vi "calcReturnTime.vi"(3 "Galvo obj array":refnum<class "Galvonometer.lvclass">[](array[class])=[refnum, refnum], 4 "Scan in":refnum<class "Scan.lvclass">, 5 "Camera in":refnum<class "Camera.lvclass">) -> (1 "Delay A":dbl, 2 "Inactive A":dbl)   [LabVIEW 2017]
uses:
  classes/Scans/Scan.lvclass
  classes/HardwareObjects/Camera/Camera.lvclass
  classes/HardwareObjects/Galvonometer/Galvonometer.lvclass
  classes/Scans/Scan.lvclass/Scan.ctl
  classes/HardwareObjects/Camera/Camera.lvclass/Camera.ctl
  classes/HardwareObjects/Galvonometer/Galvonometer.lvclass/Galvonometer.ctl
  classes/HardwareObjects/Galvonometer/Read Output Scale Factor (V_degrees).vi
  classes/HardwareObjects/Galvonometer/Read Max Scan Angle (degrees).vi
  classes/HardwareObjects/Camera/Read Max Frequency (kHz).vi
  classes/Scans/Read Scan Angle (degrees).vi
  classes/Scans/Read X FOV (degrees).vi
  classes/Scans/Read Y FOV (degrees).vi
  classes/Scans/Read Bidirectional.vi
panel:
  out "Return distance (°)":dbl=5.830951894845301
  out "Return time (s)":dbl
  out "Max angular velocity (°/s)":i32=8750
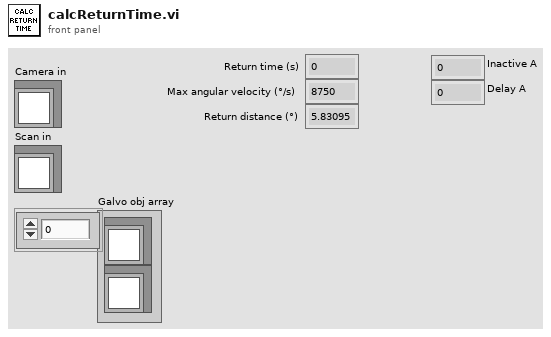
[diagram p1: front panel]
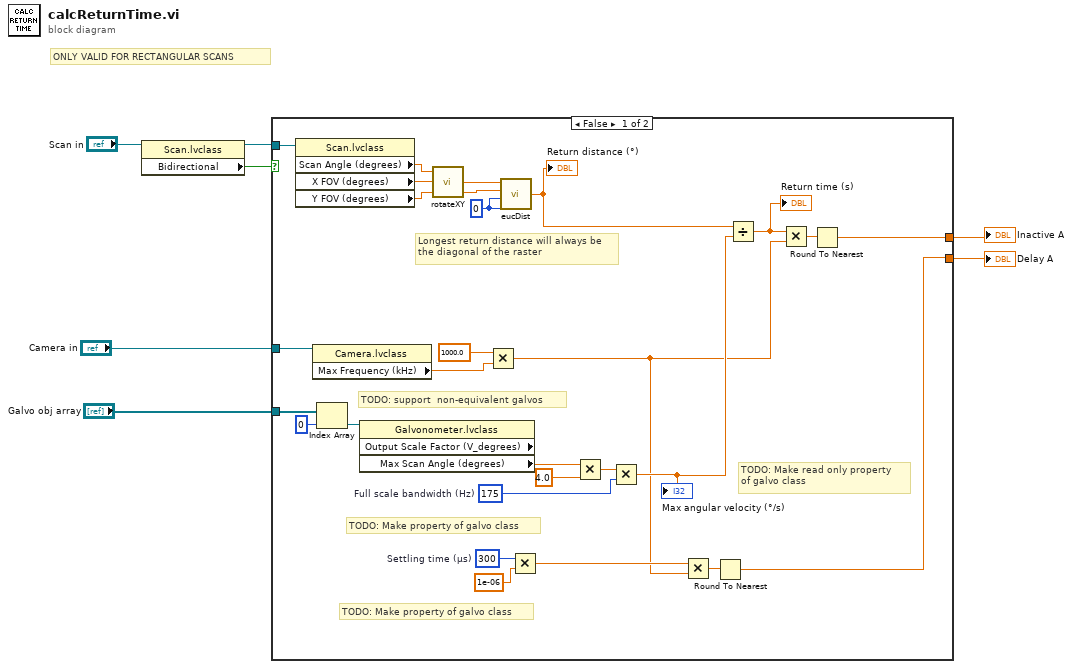
[diagram p0: block diagram]
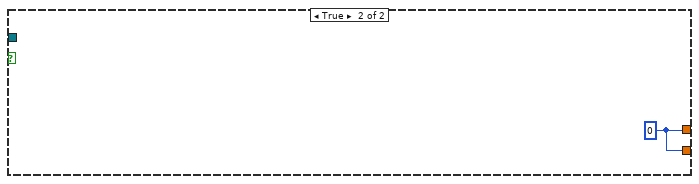
[diagram p2: hidden frame]
diagram:
  # "ONLY VALID FOR RECTANGULAR SCANS"
  n1 = property class="Scan.lvclass"(reference="Scan in") -> (reference out=w5:refnum<class "Scan.lvclass">, "Bidirectional"=w6:bool)  [unwired: 1 in, 1 out]
  n2 = case shown="False" w6 {
    tunnel: w5 -> [w35 _]
    tunnel: "Camera in" -> [w32 _]
    tunnel: "Galvo obj array" -> [w21 _]
    tunnel: [w16 w36] -> w2
    tunnel: [w15 w36] -> w1
    frame False {
      w9 = 0
      w25 = 300  # Settling time (µs)
      w22 = 175  # Full scale bandwidth (Hz)
      # "Longest return distance will always be\nthe diagonal of the raster"
      # "TODO: support  non-equivalent galvos"
      # "TODO: Make read only property\nof galvo class"
      # "TODO: Make property of galvo class"
      # "TODO: Make property of galvo class"
      # "Include safe return trip after each frame"
      n3 = property class="Scan.lvclass"(reference=w35) -> ("Scan Angle (degrees)"=w14:dbl, "X FOV (degrees)"=w13:dbl, "Y FOV (degrees)"=w12:dbl)  [unwired: 1 in, 2 out]
      n4 = property class="Camera.lvclass"(reference=w32) -> ("Max Frequency (kHz)"=w33:sgl)  [unwired: 1 in, 2 out]
      n5 = Index Array(array=w21, index=0) -> (element=w30:refnum<class "Galvonometer.lvclass">)
      n6 = property class="Galvonometer.lvclass" props=["Output Scale Factor (V_degrees)", "Max Scan Angle (degrees)"](reference=w30) -> ("Max Scan Angle (degrees)"=w29:dbl)  [unwired: 1 in, 3 out]
      n7 = call "rotateXY.vi"("B"=w12, "A"=w13, "theta"=w14) -> ("Y"=w10:dbl, "X"=w11:dbl)  [unwired: 1 in]
      n8 = Multiply(x=1000.0 ("y"), y=w33) -> (x*y=w18:dbl)
      n9 = call "eucDist.vi"("y2"=w9, "x2"=w9, "y1"=w10, "x1"=w11) -> ("d"=w8:dbl)
      "Return distance (°)" <- w8
      n10 = Multiply(x=w25, y=1e-06) -> (x*y=w24:dbl)
      n11 = Multiply(x=w29, y=4.0) -> (x*y=w28:dbl)
      n12 = Multiply(x=w28, y=w22) -> (x*y=w20:dbl)
      "Max angular velocity (°/s)" <- w20
      n13 = Multiply(x=w24, y=w18) -> (x*y=w23:dbl)
      n14 = Round To Nearest(number=w23) -> (nearest integer value=w15:dbl)
      n15 = Divide(x=w8, y=w20) -> (x/y=w19:dbl)
      "Return time (s)" <- w19
      n16 = Multiply(x=w19, y=w18) -> (x*y=w17:dbl)
      n17 = Round To Nearest(number=w17) -> (nearest integer value=w16:dbl)
    }
    frame True {
      w36 = 0
      # "No need"
    }
  }
  "Inactive A" <- w2
  "Delay A" <- w1
